vi "Main.vi"(11 "Module Admin":refnum<class "Delacor_lib_QMH_Module Admin.lvclass">) -> ()   [LabVIEW 2021, in "Model.lvlib"]
doc: "This template is based off of the Queued Message Handler design pattern and the Queued Message Handler project template that ships with LabVIEW.\n\nThe main difference is that the queue is private to this module and communication between modules is performed via Broadcast and Request events.\n\nRequest events are wrapped in public API methods and are handled in the Event Handling Loop (EHL) of this VI. Any module can register for Broadcast events sent by this module. The EHL generates messages based on user interface actions.\n\nThe Message Handling Loop (MHL) processes messages generated by the EHL, or by other messages. The messages are string values, so new messages can be added easily to the Message Cases case structure in the MHL. Each message cluster can also provide an optional value for Message Data, which is a variant that can be converted to whatever message-specific data is required.\n_____\nBased on Delacor QMH Project Template 5.0.0.82.\n\n<b>Note:</b> This VI was modified by the <b>Validate DQMH Module</b> tool to add a 'Panel Hidden' status updated broadcast to the Panel Close? event when External Launch = TRUE.\n\n<b>Note:</b> This VI was modified by the <b>Validate DQMH Module</b> tool to add a call to the Error Reported VI at the end of the 'Exit' MHL frame.\n\n<b>Note:</b> This VI was modified by the <b>Validate DQMH Module</b> tool to wrap the FP.Open method in the module close code with a Conditional Disable Structure so it does not execute when the Main VI is running as a built EXE."
uses:
  Model.lvlib
  <vilib>/Delacor/Delacor QMH/Libraries/Module Admin_class/Delacor_lib_QMH_Module Admin.lvclass
  Module Data--cluster.ctl
  <vilib>/Delacor/Delacor QMH/Libraries/Message Queue_class/Delacor_lib_QMH_Message Queue.lvclass/Delacor_lib_QMH_Message Queue.ctl
  Stop Argument--cluster.ctl
  <vilib>/Delacor/Delacor QMH/Libraries/Module Admin_class/Delacor_lib_QMH_Module Admin.lvclass/Delacor_lib_QMH_Module Admin.ctl
  Simulation Argument--cluster.ctl
  <vilib>/Utility/miscctls.llb/LVPointTypeDef.ctl
  <vilib>/Delacor/Delacor QMH/Libraries/Message Queue_class/Delacor_lib_QMH_Enqueue Message (Single).vi
  <vilib>/Delacor/Delacor QMH/Libraries/Module Admin_class/Delacor_lib_QMH_Get External Launch.vi
  <vilib>/Utility/error.llb/Error Cluster From Error Code.vi
  <vilib>/ErrorRing/Error Ring.xnode
  <vilib>/Delacor/Delacor QMH/Libraries/Message Queue_class/Delacor_lib_QMH_Message Queue.lvclass
  PS/PS.lvlib
  SCOPE/SCOPE.lvlib
  DAQ/DAQ.lvlib
panel:
  in  "SCOPE Trig":bool
  in  "DAQ Trig":bool
  in  "PS Trig":bool
  out "ModuleName":string
  out "Sim?":bool
  in  "Simulate MHL Error":bool
  in  "Simulate EHL Error":bool
  out "error out":errorcluster
  out "Status":string
  # "Instrument Panel"
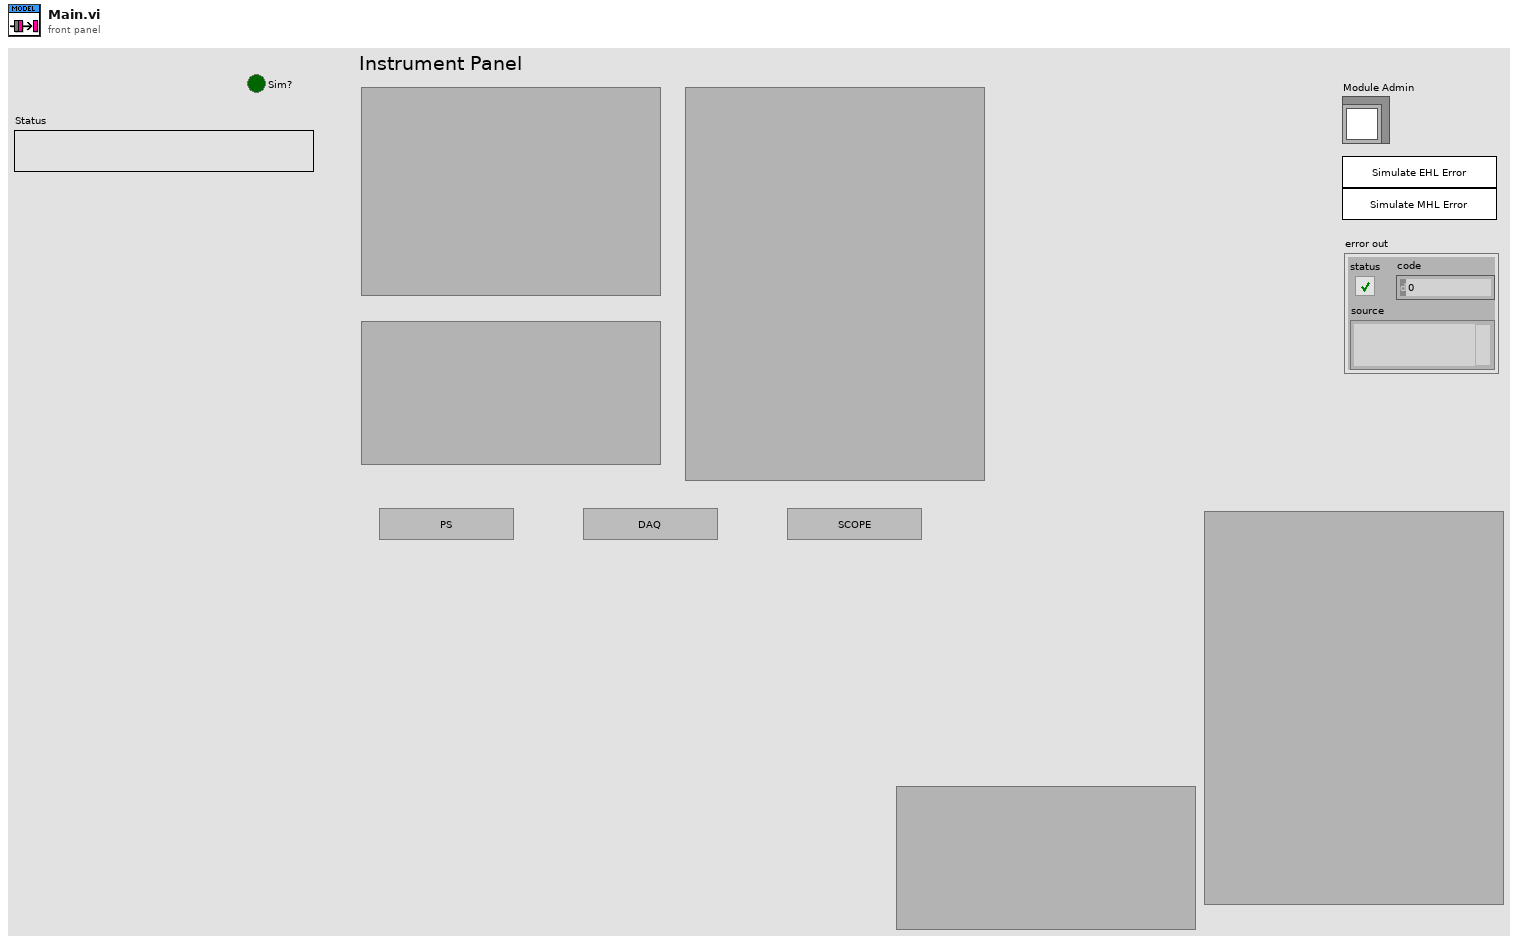
[diagram p1: front panel]
types:
  T1 = typedef "Model.lvlib/Request Events--cluster.ctl" = cluster{"Stop Module":refnum<user-event>, "Show Panel":refnum<user-event>, "Hide Panel":refnum<user-event>, "Get Module Execution Status":refnum<user-event>, "Show Diagram":refnum<user-event>, "Simulation":refnum<user-event>}
  T2 = typedef "Model.lvlib/Broadcast Events--cluster.ctl" = cluster{"Module Did Init":refnum<user-event>, "Status Updated":refnum<user-event>, "Error Reported":refnum<user-event>, "Module Did Stop":refnum<user-event>, "Update Module Execution Status":refnum<user-event>}
  T3 = typedef "PS.lvlib/Broadcast Events--cluster.ctl" = cluster{"Module Did Init":refnum<user-event>, "Status Updated":refnum<user-event>, "Error Reported":refnum<user-event>, "Module Did Stop":refnum<user-event>, "Update Module Execution Status":refnum<user-event>}
  T4 = typedef "DAQ.lvlib/Broadcast Events--cluster.ctl" = cluster{"Module Did Init":refnum<user-event>, "Status Updated":refnum<user-event>, "Error Reported":refnum<user-event>, "Module Did Stop":refnum<user-event>, "Update Module Execution Status":refnum<user-event>}
  T5 = typedef "SCOPE.lvlib/Broadcast Events--cluster.ctl" = cluster{"Module Did Init":refnum<user-event>, "Status Updated":refnum<user-event>, "Error Reported":refnum<user-event>, "Module Did Stop":refnum<user-event>, "Update Module Execution Status":refnum<user-event>}
  T6 = typedef "Model.lvlib/Module Data--cluster.ctl" = cluster{"Status":string, "Sim":bool}
  T7 = enum32{"invalid lock state", "Not Locked", "Locked (No Password)", "Password-protected"}
  T8 = typedef "Model.lvlib/Stop Argument--cluster.ctl" = cluster{"Origin":string, "Exit via Stop Module Req?":bool, "Wait for Module to stop?":bool}
  T9 = typedef "Model.lvlib/Simulation Argument--cluster.ctl" = cluster{"Sim?":bool}
  T10 = typedef "LVPointTypeDef.ctl" = cluster{"Horizontal":i16, "Vertical":i16}
  T11 = enum32{"Invalid", "Standard", "Closed", "Hidden", "Minimized", "Maximized"}
  T12 = typedef "eventvkey.ctl" = enum16{"ASCII", "Enter", "Return", "Shift", "Ctrl", "Alt", "Cmd", "Opt", "Caps", "NumLock", "Clear", "Break", "Up", "Down", "Left", "Right", "Insert", "Delete", "Home", "End", "PageUp", "PageDown", "Escape", "Help", "Pause", "ScrollLock", "F1", "F2", "F3", "F4", "F5", "F6", "F7", "F8", "F9", "F10", "F11", "F12", "F13", "F14", "F15", "F16", "F17", "F18", "F19", "F20", "F21", "F22", "F23", "F24", "Play", "VolumeUp", "VolumeDown", "Mute", "Two Byte Char"}
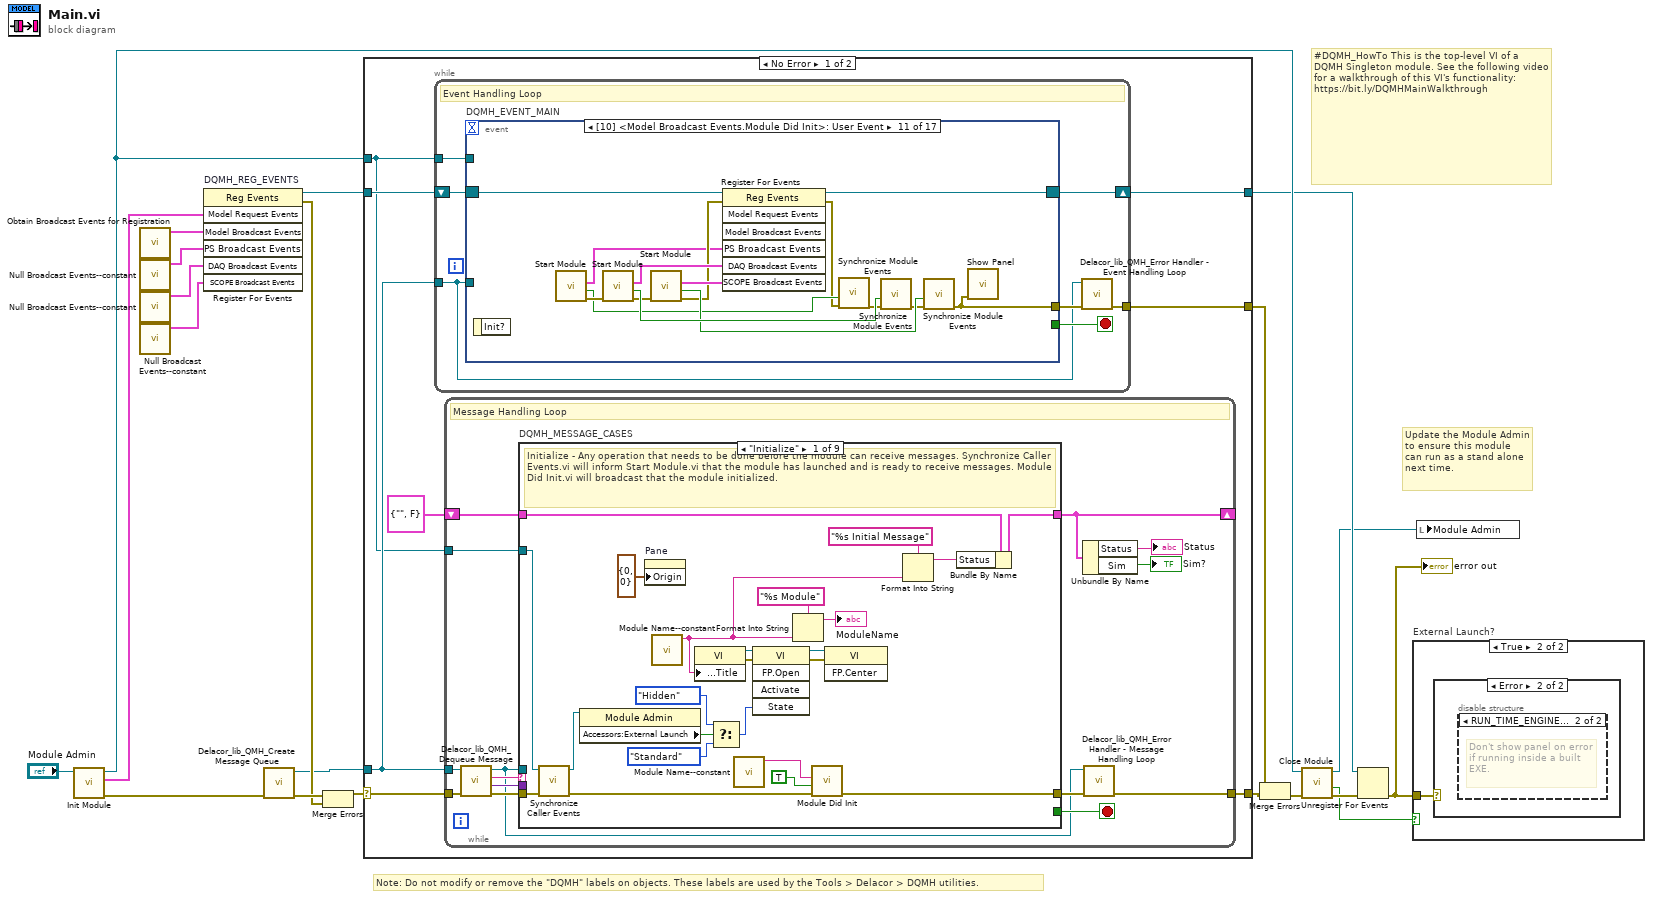
[diagram p0: block diagram]
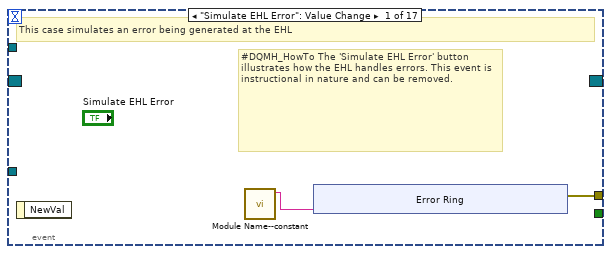
[diagram p2: hidden frame]
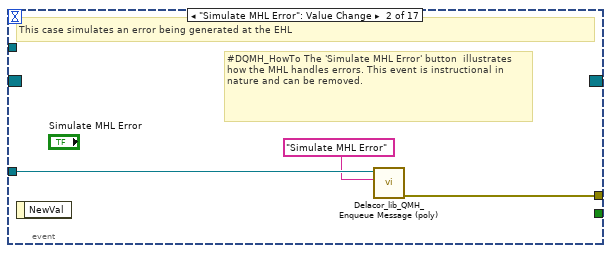
[diagram p3: hidden frame]
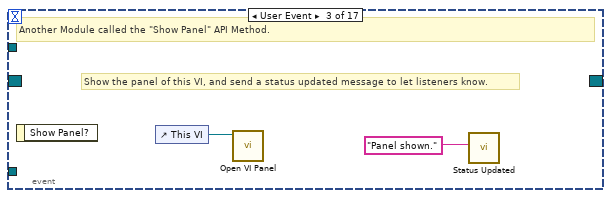
[diagram p4: hidden frame]
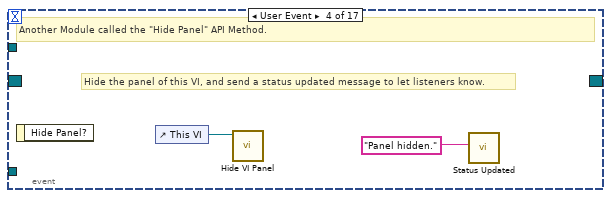
[diagram p5: hidden frame]
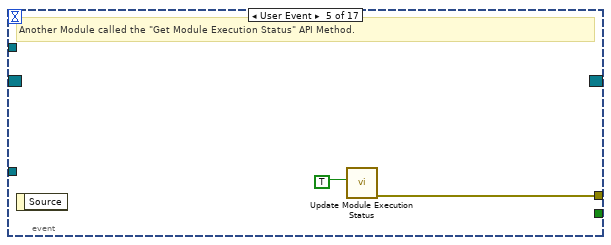
[diagram p6: hidden frame]
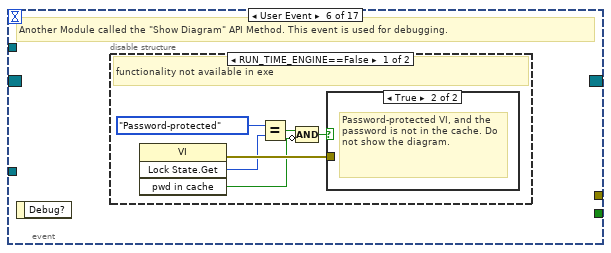
[diagram p7: hidden frame]
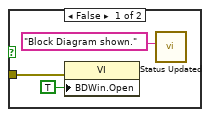
[diagram p8: hidden frame]
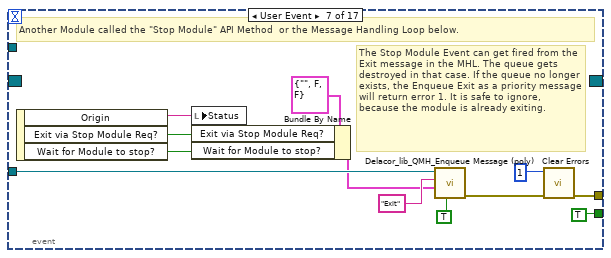
[diagram p10: hidden frame]
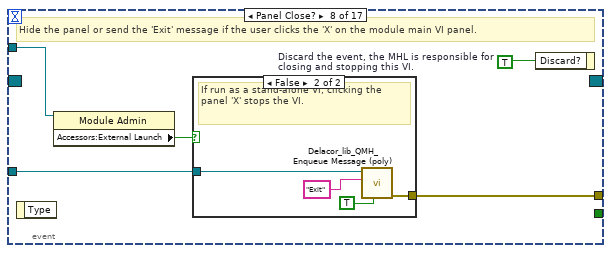
[diagram p11: hidden frame]
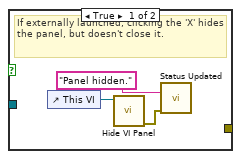
[diagram p12: hidden frame]
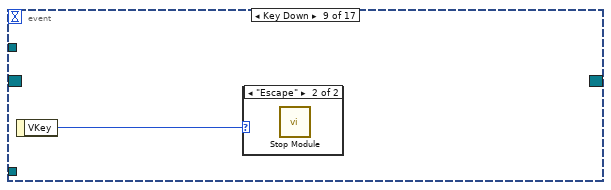
[diagram p13: hidden frame]
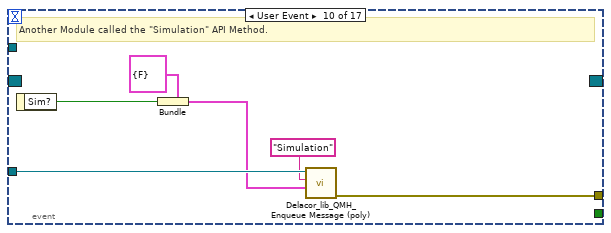
[diagram p15: hidden frame]
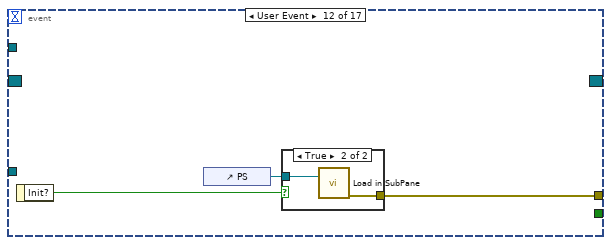
[diagram p16: hidden frame]
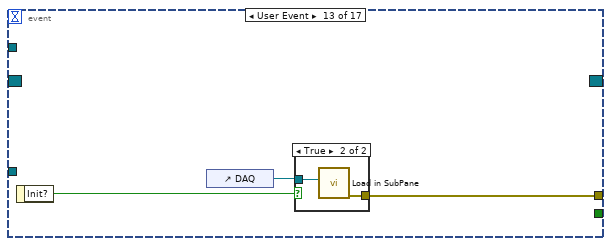
[diagram p18: hidden frame]
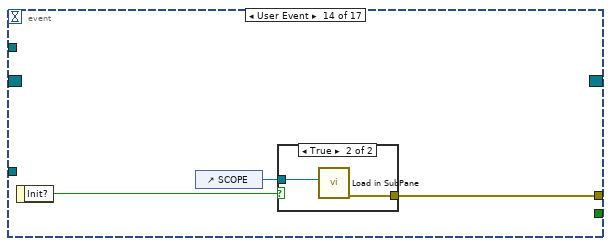
[diagram p20: hidden frame]
diagram:
  # "#DQMH_HowTo This is the top-level VI of a DQMH Singleton module. See the following video for a walkthrough of this VI's functionality: https://bit.ly/DQMHMainWalkthrough"
  # "Note: Do not modify or remove the \"DQMH\" labels on objects. These labels are used by the Tools > Delacor > DQMH utilities."
  # "Update the Module Admin to ensure this module can run as a stand alone next time."
  n1 = call "Init Module.vi"("Singleton Module Admin in"="Module Admin") -> ("error out"=w20:errorcluster, "Model Request Events"=w9:T1, "Singleton Module Admin out"=w12:refnum<class "Delacor_lib_QMH_Module Admin.lvclass">)  [unwired: 8 in]
  n2 = call "Obtain Broadcast Events for Registration.vi"() -> ("Model Broadcast Events"=w5:T2)  [unwired: 9 in, 2 out]
  n3 = call "Null Broadcast Events--constant.vi"() -> ("PS Broadcast Events"=w4:T3)  [unwired: 11 in]
  n4 = call "Null Broadcast Events--constant.vi"() -> ("DAQ Broadcast Events"=w3:T4)  [unwired: 11 in]
  n5 = call "Null Broadcast Events--constant.vi"() -> ("SCOPE Broadcast Events"=w2:T5)  [unwired: 11 in]
  n6 = register-events "DQMH_REG_EVENTS"(w9, w5, w4, w3, w2) -> (reference out=w10:refnum<event-registration>, error out=w13:errorcluster)  [unwired: 2 in]
  n7 = call <vilib>:"Delacor_lib_QMH_Create Message Queue.vi"("error in"=w20) -> ("error out"=w15:errorcluster, "Message Queue"=w8:refnum<class "Delacor_lib_QMH_Message Queue.lvclass">)  [unwired: 9 in]
  n8 = Merge Errors(w15, w13) -> (w14:errorcluster)
  n9 = case shown="No Error" w14 {
    selector: w14 -> [w27 w267]
    tunnel: [w29 w266] -> w21
    tunnel: [w26 w272] -> w11
    tunnel: w10 -> [w24 w272]
    tunnel: w8 -> [w23 w265]
    tunnel: [w28 _] -> w18
    tunnel: w12 -> [w22 w268]
    frame No Error {
      n10 = while {
        tunnel: w23 -> [w30]
        shift-right: [w33] -> w26
        shift-left: w24 -> [w34]
        tunnel: [w35] -> w28
        tunnel: w22 -> [w31]
        stop <- w32 stop-if-true
        # "Event Handling Loop"
        n11 = event "DQMH_EVENT_MAIN" shown="[10] <Model Broadcast Events.Module Did Init>: User Event" {
          selector: w34 -> [_ _ _ _ _ _ _ _ _ _ w109 _ _ _ _ _ _]
          dyn-events: [_ _ _ _ _ _ _ _ _ _ w108 _ _ _ _ _ _] -> w33
          timeout: _ -> [_ _ _ _ _ _ _ _ _ _ _ _ _ _ _ _ _]
          tunnel: [_ _ _ _ _ _ TRUE ("Discard?") _ _ _ _ _ _ _ _ _ _] -> w32
          tunnel: w30 -> [_ w47 _ _ _ _ w71 w78 _ w94 _ _ _ _ _ _ _]
          tunnel: [w38 w48 _ _ w54 _ w74 w80 _ w89 w100 w112 w117 w122 w127 w132 w139] -> w36
          tunnel: w31 -> [_ _ _ _ _ _ _ w77 _ _ _ _ _ _ _ _ _]
          event "Simulate EHL Error": Value Change {
            # "#DQMH_HowTo The 'Simulate EHL Error' button  illustrates how the EHL handles errors. This event is instructional in nature and can be removed."
            # "This case simulates an error being generated at the EHL"
            n12 = event-data() -> ()  [unwired: 1 in, 1 out]
            n13 = call "Module Name--constant.vi"() -> ("Module Name"=w37:string)  [unwired: 11 in]
            n14 = xnode ("Error Ring")("parameter 0"=w37) -> ("error out"=w38:errorcluster)
          }
          event "Simulate MHL Error": Value Change {
            # "#DQMH_HowTo The 'Simulate MHL Error' button  illustrates how the MHL handles errors. This event is instructional in nature and can be removed."
            # "This case simulates an error being generated at the EHL"
            n15 = event-data() -> ()  [unwired: 1 in, 1 out]
            n16 = call-poly <vilib>:"Delacor_lib_QMH_Enqueue Message (poly).vi"("Message"="Simulate MHL Error", "Message Queue in"=w47) -> ("error out"=w48:errorcluster)  [unwired: 8 in, 1 out]
          }
          event User Event {
            # "Show the panel of this VI, and send a status updated message to let listeners know."
            # "Another Module called the \"Show Panel\" API Method."
            n17 = event-data() -> ()  [unwired: 1 in, 1 out]
            n18 = control-ref of="This VI"() -> (w50:refnum<vi>)
            n19 = call "Open VI Panel.vi"("VI"=w50) -> ()  [unwired: 10 in, 1 out]
            n20 = call "Status Updated.vi"("Status"="Panel shown." ("format string")) -> ()  [unwired: 10 in, 1 out]
          }
          event User Event {
            # "Hide the panel of this VI, and send a status updated message to let listeners know."
            # "Another Module called the \"Hide Panel\" API Method."
            n21 = event-data() -> ()  [unwired: 1 in, 1 out]
            n22 = control-ref of="This VI"() -> (w52:refnum<vi>)
            n23 = call "Hide VI Panel.vi"("VI"=w52) -> ()  [unwired: 10 in, 1 out]
            n24 = call "Status Updated.vi"("Status"="Panel hidden." ("format string")) -> ()  [unwired: 10 in, 1 out]
          }
          event User Event {
            # "Another Module called the \"Get Module Execution Status\" API Method."
            n25 = event-data() -> ()  [unwired: 1 in, 1 out]
            n26 = call "Update Module Execution Status.vi"("Running?"=TRUE) -> ("error out"=w54:errorcluster)  [unwired: 10 in]
          }
          event User Event {
            # "Another Module called the \"Show Diagram\" API Method. This event is used for debugging."
            n27 = event-data() -> ()  [unwired: 1 in, 1 out]
            n28 = disable-structure "Conditional Disable Structure" shown="RUN_TIME_ENGINE==False" {
              frame condition #0 (active) {
                # "functionality not available in exe"
                n29 = invoke on="Invoke Node" class="VI" method="Lock State.Get"() -> (error out=w60:errorcluster, "Get Lock State"=w59:T7, "pwd in cache"=w56:bool)  [unwired: 4 in, 1 out]
                n30 = Equal?(x=T7."Password-protected", y=w59) -> (x = y?=w57:bool)
                n31 = Compound Arithmetic op=AND(w57, invert w56) -> (w55:bool)
                n32 = case shown="True" w55 {
                  tunnel: w60 -> [w63 _]
                  frame False {
                    n33 = property on="Property Node" class="VI"(error in=w63, "BDWin.Open"=TRUE ("Block Diagram Window:Open")) -> ()  [unwired: 1 in, 2 out]
                    n34 = call "Status Updated.vi"("Status"="Block Diagram shown." ("format string")) -> ()  [unwired: 10 in, 1 out]
                  }
                  frame True {
                    # "Password-protected VI, and the password is not in the cache. Do not show the diagram."
                  }
                }
              }
              frame condition #1 {
              }
            }
          }
          event User Event {
            # "The Stop Module Event can get fired from the Exit message in the MHL. The queue gets destroyed in that case. If the queue no longer exists, the Enqueue Exit as a priority message will return error 1. It is safe to ignore, because the module is already exiting."
            # "Another Module called the \"Stop Module\" API Method  or the Message Handling Loop below."
            n35 = event-data() -> ("Origin"=w70:string, "Exit via Stop Module Req?"=w66:bool, "Wait for Module to stop?"=w65:bool)  [unwired: 1 in]
            n36 = local write "Status"(w70) -> ()
            n37 = Bundle By Name(cluster=T8 {"Origin"="", "Exit via Stop Module Req?"=FALSE, "Wait for Module to stop?"=FALSE} ("Stop Argument"), "Exit via Stop Module Req?"=w66, "Wait for Module to stop?"=w65) -> (w64:T8)
            n38 = call-poly <vilib>:"Delacor_lib_QMH_Enqueue Message (poly).vi"("Priority Message? (F)"=TRUE, "Message Data"=w64, "Message"="Exit", "Message Queue in"=w71) -> ("error out"=w75:errorcluster)  [unwired: 6 in, 1 out]
            n39 = call <vilib>:"Clear Errors.vi"("error in (no error)"=w75, "specific error code to clear (0: all)"=1) -> ("error out"=w74:errorcluster)  [unwired: 4 in, 1 out]
          }
          event Panel Close? {
            w79 = TRUE  # Discard the event, the MHL is responsible for closing and stopping this VI.
            # "Hide the panel or send the 'Exit' message if the user clicks the 'X' on the module main VI panel."
            n40 = event-data() -> ()  [unwired: 1 in, 1 out]
            n41 = property on="Property Node" class="Module Admin"(reference=w77) -> ("Accessors:External Launch"=w76:bool)  [unwired: 1 in, 2 out]
            n42 = case shown="False" w76 {
              tunnel: w78 -> [_ w86]
              tunnel: [_ w87] -> w80
              frame True {
                # "If externally launched, clicking the 'X' hides the panel, but doesn't close it."
                n43 = control-ref of="This VI"() -> (w83:refnum<vi>)
                n44 = call "Hide VI Panel.vi"("VI"=w83) -> ("error out"=w81:errorcluster)  [unwired: 10 in]
                n45 = call "Status Updated.vi"("error in (no error)"=w81, "Status"="Panel hidden.") -> ()  [unwired: 9 in, 1 out]
              }
              frame False {
                # "If run as a stand-alone VI, clicking the panel 'X' stops the VI."
                n46 = call-poly <vilib>:"Delacor_lib_QMH_Enqueue Message (poly).vi"("Priority Message? (F)"=TRUE, "Message"="Exit", "Message Queue in"=w86) -> ("error out"=w87:errorcluster)  [unwired: 7 in, 1 out]
              }
            }
            n47 = event-data ("Event Filter Node")("Discard?"=w79) -> ()  [unwired: 1 in, 1 out]
          }
          event Key Down {
            n48 = event-data() -> ("VKey"=w88:T12)  [unwired: 1 in]
            n49 = case shown="\"Escape\"" w88 {
              frame "ASCII", Default {
              }
              frame "Escape" {
                n50 = call "Stop Module.vi"() -> ()  [unwired: 11 in, 1 out]
              }
            }
          }
          event User Event {
            # "Another Module called the \"Simulation\" API Method."
            n51 = event-data() -> ("Sim?"=w90:bool)  [unwired: 1 in]
            n52 = Bundle(cluster=T9 {"Sim?"=FALSE} ("Simulation Argument"), "Sim?"=w90) -> (w91:T9)
            n53 = call-poly <vilib>:"Delacor_lib_QMH_Enqueue Message (poly).vi"("Message Data"=w91, "Message"="Simulation", "Message Queue in"=w94) -> ("error out"=w89:errorcluster)  [unwired: 7 in, 1 out]
          }
          event User Event {
            n54 = event-data() -> ()  [unwired: 1 in, 1 out]
            n55 = call "Start Module.vi"() -> ("error out"=w99:errorcluster, "Wait for Event Sync?"=w97:bool, "PS Broadcast Events"=w95:T3)  [unwired: 7 in, 2 out]
            n56 = call "Start Module.vi"("error in (no error)"=w99) -> ("error out"=w103:errorcluster, "Wait for Event Sync?"=w107:bool, "SCOPE Broadcast Events"=w105:T5)  [unwired: 6 in, 2 out]
            n57 = call "Start Module.vi"("error in (no error)"=w103) -> ("error out"=w102:errorcluster, "Wait for Event Sync?"=w106:bool, "DAQ Broadcast Events"=w104:T4)  [unwired: 6 in, 2 out]
            n58 = register-events(reference=w109, error in=w102, w95, w105, w104) -> (reference out=w108:refnum<event-registration>, error out=w96:errorcluster)  [unwired: 2 in]
            n59 = call "Synchronize Module Events.vi"("error in (no error)"=w96, "Wait for Event Sync?"=w97) -> ("error out"=w98:errorcluster)  [unwired: 9 in]
            n60 = call "Synchronize Module Events.vi"("error in (no error)"=w98, "Wait for Event Sync?"=w107) -> ("error out"=w101:errorcluster)  [unwired: 9 in]
            n61 = call "Synchronize Module Events.vi"("error in (no error)"=w101, "Wait for Event Sync?"=w106) -> ("error out"=w100:errorcluster)  [unwired: 9 in]
            n62 = call "Show Panel.vi"("error in (no error)"=w100) -> ()  [unwired: 10 in, 1 out]
          }
          event User Event {
            n63 = event-data() -> ("Init?"=w111:bool)  [unwired: 1 in]
            n64 = control-ref of="PS"() -> (w110:refnum<vi>)
            n65 = case shown="True" w111 {
              tunnel: [_ w114] -> w112
              tunnel: w110 -> [_ w113]
              frame False {
              }
              frame True {
                n66 = call "Load in SubPane.vi"("Subpanel Ref"=w113) -> ("error out"=w114:errorcluster)  [unwired: 10 in]
              }
            }
          }
          event User Event {
            n67 = event-data() -> ("Init?"=w116:bool)  [unwired: 1 in]
            n68 = control-ref of="DAQ"() -> (w115:refnum<vi>)
            n69 = case shown="True" w116 {
              tunnel: [_ w119] -> w117
              tunnel: w115 -> [_ w118]
              frame False {
              }
              frame True {
                n70 = call "Load in SubPane.vi"("Subpanel Ref"=w118) -> ("error out"=w119:errorcluster)  [unwired: 10 in]
              }
            }
          }
          event User Event {
            n71 = event-data() -> ("Init?"=w121:bool)  [unwired: 1 in]
            n72 = control-ref of="SCOPE"() -> (w120:refnum<vi>)
            n73 = case shown="True" w121 {
              tunnel: [_ w124] -> w122
              tunnel: w120 -> [_ w123]
              frame False {
              }
              frame True {
                n74 = call "Load in SubPane.vi"("Subpanel Ref"=w123) -> ("error out"=w124:errorcluster)  [unwired: 10 in]
              }
            }
          }
          event "PS Trig": Value Change {
            n75 = event-data() -> ("NewVal"=w126:bool)  [unwired: 1 in]
            n76 = control-ref of="PS"() -> (w125:refnum<vi>)
            n77 = case shown="True" w126 {
              tunnel: [w129 w130] -> w127
              tunnel: w125 -> [w128 w131]
              frame False {
                n78 = call "UnLoad SubPane.vi"("Subpanel Ref"=w128) -> ("error out"=w129:errorcluster)  [unwired: 10 in]
              }
              frame True {
                n79 = call "Load in SubPane.vi"("Subpanel Ref"=w131) -> ("error out"=w130:errorcluster)  [unwired: 10 in]
              }
            }
          }
          event "DAQ Trig": Value Change {
            n80 = event-data() -> ("NewVal"=w134:bool)  [unwired: 1 in]
            n81 = control-ref of="DAQ"() -> (w133:refnum<vi>)
            n82 = case shown="True" w134 {
              tunnel: w133 -> [w136 w138]
              tunnel: [w135 w137] -> w132
              frame False {
                n83 = call "UnLoad SubPane.vi"("Subpanel Ref"=w136) -> ("error out"=w135:errorcluster)  [unwired: 10 in]
              }
              frame True {
                n84 = call "Load in SubPane.vi"("Subpanel Ref"=w138) -> ("error out"=w137:errorcluster)  [unwired: 10 in]
              }
            }
          }
          event "SCOPE Trig": Value Change {
            n85 = event-data() -> ("NewVal"=w141:bool)  [unwired: 1 in]
            n86 = control-ref of="SCOPE"() -> (w140:refnum<vi>)
            n87 = case shown="True" w141 {
              tunnel: w140 -> [w143 w145]
              tunnel: [w142 w144] -> w139
              frame False {
                n88 = call "UnLoad SubPane.vi"("Subpanel Ref"=w143) -> ("error out"=w142:errorcluster)  [unwired: 10 in]
              }
              frame True {
                n89 = call "Load in SubPane.vi"("Subpanel Ref"=w145) -> ("error out"=w144:errorcluster)  [unwired: 10 in]
              }
            }
          }
        }
        n90 = call-dynamic "Delacor_lib_QMH_Error Handler - Event Handling Loop.vi"("error in"=w36, "Message Queue in"=w30) -> ("dup error in"=w35:errorcluster)  [unwired: 8 in, 1 out]
      }
      n91 = while {
        tunnel: w23 -> [w151]
        shift-right: [w148] -> _
        shift-left: T6 {"Status"="", "Sim"=FALSE} ("Data Cluster") -> [w155]
        tunnel: w27 -> [w158]
        tunnel: [w156] -> w29
        tunnel: w22 -> [w149]
        stop <- w154 stop-if-true
        # "Message Handling Loop"
        n92 = call-dynamic "Delacor_lib_QMH_Dequeue Message.vi"("error in"=w158, "Message Queue in"=w151) -> ("error out"=w157:errorcluster, "Message Data"=w152:variant, "Message"=w153:string, "Message Queue out"=w150:refnum<class "Delacor_lib_QMH_Message Queue.lvclass">)  [unwired: 6 in]
        n93 = case "DQMH_MESSAGE_CASES" shown="\"Initialize\"" w153 {
          selector: w153 -> [_ _ w191 _ _ _ _ _ w252]
          tunnel: w150 -> [_ _ _ _ _ _ w218 w245 _]
          tunnel: w157 -> [w180 w184 w198 w201 w203 w208 w225 w250 w254]
          tunnel: [w178 w184 w196 w200 w203 w207 w221 w247 w255] -> w159
          tunnel: w155 -> [w170 w183 w197 w199 w202 w205 w220 w244 w253]
          tunnel: [w169 w183 w192 w199 w202 w205 w220 w244 w253] -> w148
          tunnel: [_ _ _ _ _ _ _ w243 _] -> w154
          tunnel: w152 -> [_ _ w195 _ _ _ w219 w242 _]
          tunnel: w149 -> [w171 _ _ _ _ _ w217 w237 _]
          frame "Initialize" {
            # "Initialize - Any operation that needs to be done before the module can receive messages. Synchronize Caller Events.vi will inform Start Module.vi that the module has launched and is ready to receive messages. Module Did Init.vi will broadcast that the module initialized."
            n94 = call "Synchronize Caller Events.vi"("error in (no error)"=w180, "Singleton Module Admin in"=w171) -> ("error out"=w179:errorcluster, "Singleton Module Admin out"=w166:refnum<class "Delacor_lib_QMH_Module Admin.lvclass">)  [unwired: 8 in]
            n95 = property on="Property Node" class="Module Admin"(reference=w166) -> ("Accessors:External Launch"=w175:bool)  [unwired: 1 in, 2 out]
            n96 = property on="Pane" class="Pane"("Origin"=T10 {"Horizontal"=0, "Vertical"=0}) -> ()  [unwired: 2 in, 2 out]
            n97 = call "Module Name--constant.vi"() -> ("Module Name"=w162:string)  [unwired: 11 in]
            n98 = property on="Property Node" class="VI"("Front Panel.Title"=w162) -> (reference out=w177:refnum<vi>, error out=w182:errorcluster)  [unwired: 2 in]
            n99 = Select(t=T11."Hidden" ("State"), s=w175, f=T11."Standard" ("State")) -> (s? t:f=w172:T11)
            n100 = call "Module Name--constant.vi"() -> ("Module Name"=w167:string)  [unwired: 11 in]
            n101 = invoke on="Invoke Node" class="VI" method="FP.Open"(reference=w177, error in=w182, "State"=w172) -> (reference out=w176:refnum<vi>, error out=w181:errorcluster)  [unwired: 2 in, 3 out]
            n102 = Format Into String(format string="%s Module", w162) -> (resulting string=→"ModuleName":string)  [unwired: 2 in, 1 out]
            n103 = call "Module Did Init.vi"("error in (no error)"=w179, "Initialized?"=TRUE, "Origin"=w167) -> ("error out"=w178:errorcluster)  [unwired: 8 in]
            n104 = invoke on="Invoke Node" class="VI" method="FP.Center"(reference=w176, error in=w181) -> ()  [unwired: 1 in, 3 out]
            n105 = Format Into String(format string="%s Initial Message" ("Initial Message"), w162) -> (resulting string=w164:string)  [unwired: 2 in, 1 out]
            n106 = Bundle By Name(cluster=w170, "Status"=w164) -> (w169:T6)
          }
          frame "--- Module Specific ---" {
            # "Separator -- The following cases handle messages specific to this Module."
          }
          frame "Simulation" {
            # "This will change Module into Simulation Mode"
            n107 = Variant To Data(error in=w198, type=T9 {"Sim?"=FALSE} ("Simulation Argument"), Variant=w195) -> (data=w193:T9, error out=w196:errorcluster)
            n108 = Unbundle By Name(w193) -> ("Sim?"=w190:bool)
            n109 = Select(t="True", s=w190, f="False") -> (s? t:f=w186:string)
            n110 = Format Into String(format string="%s: %s", w191, w186) -> (resulting string=w185:string)  [unwired: 2 in, 1 out]
            n111 = Bundle By Name(cluster=w197, "Status"=w185, "Sim"=w190) -> (w192:T6)
          }
          frame "---Copy This Frame---" {
            # "Duplicate this frame when creating new messages.  Change this comment in the duplicated frame to describe this message."
            n112 = Merge Errors(w201) -> (w200:errorcluster)
          }
          frame "--- Exit and Error Handling---" {
            # "Separator - The following cases handle errors and exit messages."
          }
          frame "Simulate MHL Error" {
            # "#DQMH_HowTo The 'Simulate MHL Error' button  illustrates how the MHL handles errors. This event is instructional in nature and can be removed."
            # "Simulate an error occurring at the MHL"
            n113 = call "Module Name--constant.vi"() -> ("Module Name"=w204:string)  [unwired: 11 in]
            n114 = xnode ("Error Ring")("parameter 0"=w204) -> ("error out"=w206:errorcluster)
            n115 = Merge Errors(w208, w206) -> (w207:errorcluster)
          }
          frame "Error" {
            # "#CodeRecommended - If you ever change the name of this \"Error\" message, you'll need to update the name in the Check Loop Error.vi as well."
            # "#CodeRecommended - If the module is running in standalone mode (External Launch = FALSE), this code will pop up an error dialog and call the 'Exit' message if an error occurs. Add more fine-grained error handling here."
            # "Error - Check the error message data and respond accordingly. This message is sent by the \"Error Handler\" VIs at the end of each loop in this application."
            n116 = property on="Property Node" class="Module Admin"(reference=w217) -> ("Accessors:External Launch"=w216:bool)  [unwired: 1 in, 2 out]
            n117 = Variant To Data(error in=w225, type=errorcluster {"status"=FALSE, "code"=0, "source"=""} ("error constant"), Variant=w219) -> (data=w226:errorcluster, error out=w223:errorcluster)
            n118 = call "Error Reported.vi"("Error"=w226) -> ()  [unwired: 10 in, 1 out]
            n119 = case shown="False" w216 {
              tunnel: [w231 _] -> w222
              tunnel: w218 -> [w229 _]
              tunnel: w226 -> [w230 _]
              frame False {
                # "If the module is running standalone, then pop up an error dialog and call the \"Exit\" message."
                n120 = call <vilib>:"Simple Error Handler.vi"("error in (no error)"=w230) -> ()  [unwired: 4 in, 5 out]
                n121 = call-poly <vilib>:"Delacor_lib_QMH_Enqueue Message (poly).vi"("Priority Message? (F)"=TRUE, "Message"="Exit", "Message Queue in"=w229) -> ("error out"=w231:errorcluster)  [unwired: 7 in, 1 out]
              }
              frame True {
                # "If the module was launched externally, calling the Error Reported broadcast VI is the only action performed by the \"Error\" message. The module's caller can then process the error appropriately."
              }
            }
            n122 = Merge Errors(w223, w222) -> (w221:errorcluster)
            n123 = local write "error out"(w221) -> ()
          }
          frame "Exit" {
            w241 = 91  # 91: not all Exit messages will have an argument
            w243 = TRUE  # Stop the VI
            # "Release the message queue reference"
            # "Exit - Exit the application."
            n124 = Variant To Data(error in=w250, type=T8 {"Origin"="", "Exit via Stop Module Req?"=FALSE, "Wait for Module to stop?"=FALSE} ("Stop Argument"), Variant=w242) -> (data=w239:T8, error out=w246:errorcluster)
            n125 = call "Stop Module.vi"() -> ("error out"=w233:errorcluster)  [unwired: 11 in]
            n126 = call <vilib>:"Clear Errors.vi"("error in (no error)"=w246, "specific error code to clear (0: all)"=w241) -> ("error out"=w249:errorcluster)  [unwired: 4 in, 1 out]
            n127 = call "Stop Module.vi"() -> ("error out"=w234:errorcluster)  [unwired: 11 in]
            n128 = call "Stop Module.vi"() -> ("error out"=w235:errorcluster)  [unwired: 11 in]
            n129 = control-ref of="This VI"() -> (w238:refnum<vi>)
            n130 = Merge Errors(w235, w234, w233) -> (w232:errorcluster)
            n131 = call-dynamic "Delacor_lib_QMH_Release Message Queue.vi"("error in"=w249, "Message Queue"=w245) -> ("error out"=w248:errorcluster)  [unwired: 9 in]
            n132 = call "Handle Exit.vi"("error in (no error)"=w232, "Stop Argument"=w239, "Admin in"=w237, "VI reference"=w238) -> ("error out"=w236:errorcluster)  [unwired: 6 in, 1 out]
            n133 = Merge Errors(w248, w236) -> (w247:errorcluster)
            n134 = call "Error Reported.vi"("Error"=w247) -> ()  [unwired: 10 in, 1 out]
          }
          frame Default {
            # "'Default' case only runs if there is a message that isn't defined in any of the other cases.  Output a programming error."
            n135 = call "Module Name--constant.vi"() -> ("Module Name"=w251:string)  [unwired: 11 in]
            n136 = xnode ("Error Ring")("parameter 0"=w252, "parameter 1"=w251) -> ("error out"=w256:errorcluster)
            n137 = Merge Errors(w254, w256) -> (w255:errorcluster)
          }
        }
        n138 = Unbundle By Name(w148) -> ("Status"=→"Status":string, "Sim"=→"Sim?":bool)
        n139 = call-dynamic "Delacor_lib_QMH_Error Handler - Message Handling Loop.vi"("error in"=w159, "Message Queue in"=w150) -> ("dup error in"=w156:errorcluster)  [unwired: 8 in, 1 out]
      }
    }
    frame Error {
      # "Synchronize Caller Events.vi will inform Start Module.vi that the module has launched and will let the code calling Start Module.vi register for broadcasts and would permit the caller receive the broadcast that an error occurred at launch time."
      n140 = call-dynamic "Delacor_lib_QMH_Release Message Queue.vi"("error in"=w267, "Message Queue"=w265) -> ("error out"=w266:errorcluster)  [unwired: 9 in]
      n141 = call "Synchronize Caller Events.vi"("Singleton Module Admin in"=w268) -> ("error out"=w273:errorcluster)  [unwired: 9 in, 1 out]
      n142 = call "Module Name--constant.vi"() -> ("Module Name"=w271:string)  [unwired: 11 in]
      n143 = Format Into String(format string="An error occurred during initialization. %s is no longer running.", w271) -> (resulting string=w269:string)  [unwired: 2 in, 1 out]
      n144 = Merge Errors(w266, w273) -> (w274:errorcluster)
      n145 = call "Error Reported.vi"("Additional Information"=w269, "Error"=w274) -> ()  [unwired: 9 in, 1 out]
    }
  }
  n146 = Merge Errors(w18, w21) -> (w17:errorcluster)
  n147 = call "Close Module.vi"("error in (no error)"=w17, "Module Admin in"=w12) -> ("error out"=w19:errorcluster, "External Launch"=w1:bool, "Module Admin out"=w6:refnum<class "Delacor_lib_QMH_Module Admin.lvclass">)  [unwired: 7 in]
  n148 = Unregister For Events(event registration refnum=w11, error in=w19) -> (error out=w16:errorcluster)
  "error out" <- w16
  n149 = case "External Launch?" shown="True" w1 {
    tunnel: w16 -> [_ w275]
    frame False {
    }
    frame True {
      n150 = case shown="Error" w275 {
        frame No Error {
          n151 = invoke on="Invoke Node" class="VI" method="FP.Close"() -> ()  [unwired: 3 in, 3 out]
        }
        frame Error {
          n152 = disable-structure shown="RUN_TIME_ENGINE==True" {
            frame condition #0 (active) {
              n153 = invoke class="VI" method="FP.Open"("Activate"=TRUE ("Activate?")) -> ()  [unwired: 4 in, 5 out]
            }
            frame condition #1 {
              # "Don't show panel on error if running inside a built EXE."
            }
          }
        }
      }
    }
  }
  n154 = local write "Module Admin"(w6) -> ()
